vi "映射文件写入XML.vi"(8 "error in (no error)":errorcluster, 11 "project":T1) -> (0 "error out":errorcluster)   [LabVIEW 2016, in "Alarm interface.lvlib"]
uses:
  Alarm interface.lvlib
  <vilib>/Utility/xml.llb/Write to XML File(string).vi
panel:
  out "文本":string
  out "xml字符串":string
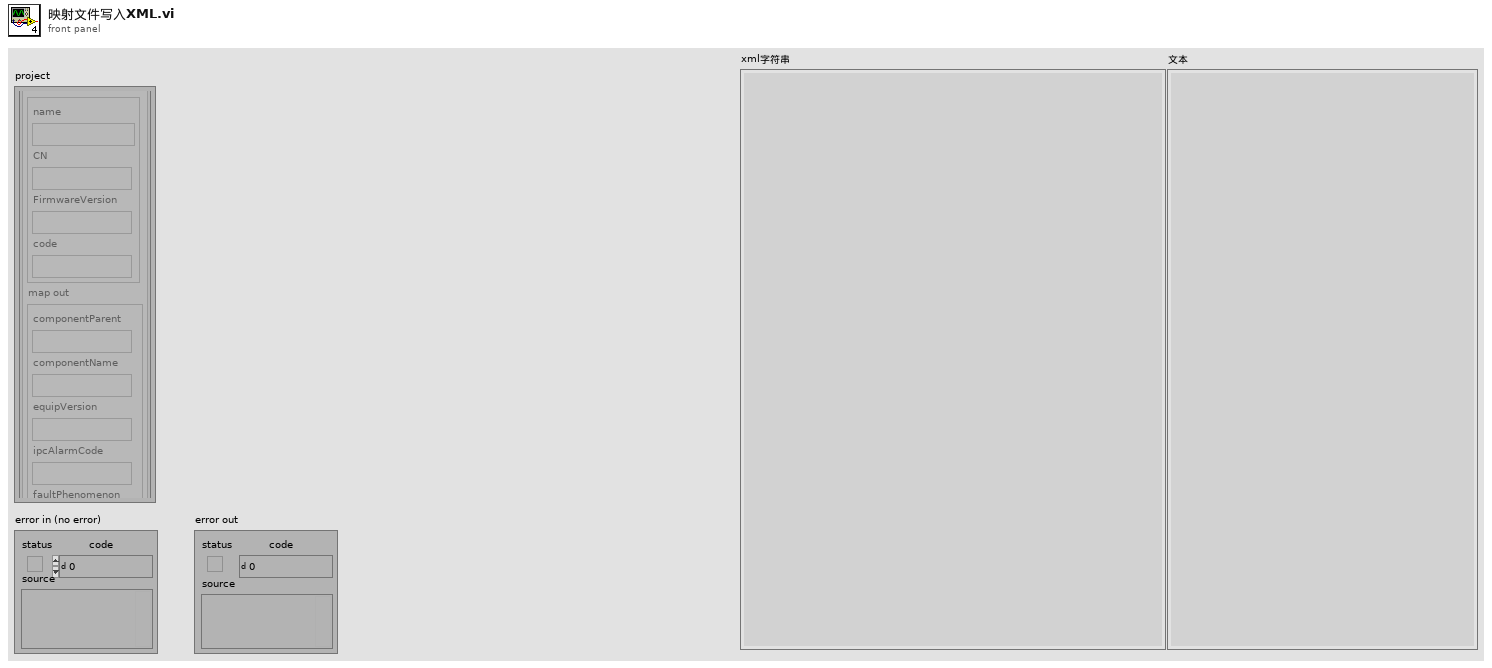
[diagram p1: front panel]
types:
  T1 = typedef "Alarm interface.lvlib/map project.ctl" = cluster{"data":T2[]}
  T2 = typedef "Alarm interface.lvlib/map data.ctl" = cluster{"map in":T3, "map out":T4}
  T3 = typedef "Alarm interface.lvlib/map in.ctl" = cluster{"name":string, "CN":string, "FirmwareVersion":string, "code":string}
  T4 = typedef "Alarm interface.lvlib/map out.ctl" = cluster{"componentParent":string, "componentName":string, "equipVersion":string, "ipcAlarmCode":string, "faultPhenomenon":string}
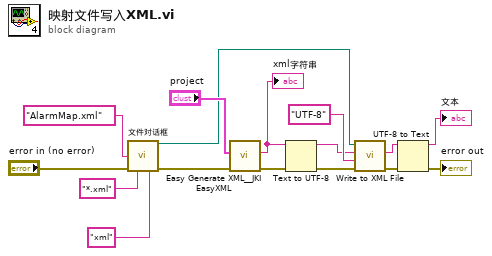
[diagram p0: block diagram]
diagram:
  n1 = call "文件对话框"("default name"="AlarmMap.xml", "error in"="error in (no error)", "pattern (all files)"="*.xml", "pattern label"="xml") -> ("selected path"=w6:path, "error out"=w1:errorcluster)  [unwired: 8 in, 2 out]
  n2 = call <vilib>:"Easy Generate XML__JKI EasyXML.vi"("error in (no error)"=w1, "LabVIEW Data"="project") -> ("error out"=w9:errorcluster, "XML String"=w14:string)  [unwired: 8 in]
  "xml字符串" <- w14
  n3 = Text to UTF-8(8:w9, 11:w14) -> (0:w8:errorcluster, 3:w13:string)  [unwired: 1 in]
  n4 = call-poly <vilib>:"Write to XML File.vi"("error in (no error)"=w8, "XML Encoding"="UTF-8", "XML Input"=w13, "XML File Path"=w6) -> ("error out"=w10:errorcluster, "XML String"=w12:string)  [unwired: 5 in, 1 out]
  n5 = UTF-8 to Text(8:w10, 11:w12) -> (0:→"error out":errorcluster, 3:→"文本":string)  [unwired: 1 in]
